vi "S2DS_Update Additional Info from user.vi"(11 "File info (in)":T1={"File path"=path "", "Header"="", "File name"="", "False channel"=[], "Channel names"=[], "Buffer size"=0, "Format"="%.6f"}) -> (2 "OK 2":bool, 3 "File info (out)":T1={"File path"=path "", "Header"="", "File name"="", "False channel"=[], "Channel names"=[], "Buffer size"=0, "Format"="%.6f"})   [LabVIEW 2025]
uses:
  TYPE DEFS/S2DS_Data saving info.ctl
panel:
  in  "CANCEL SWEEP":bool
  in  "Purpose":string
  in  "Skip":bool
  in  "OK":bool
  in  "False channel in (User)":string[][](array[string]) caption="Common information"
  # "Additional information"
  # "Information name"
  # "Value"
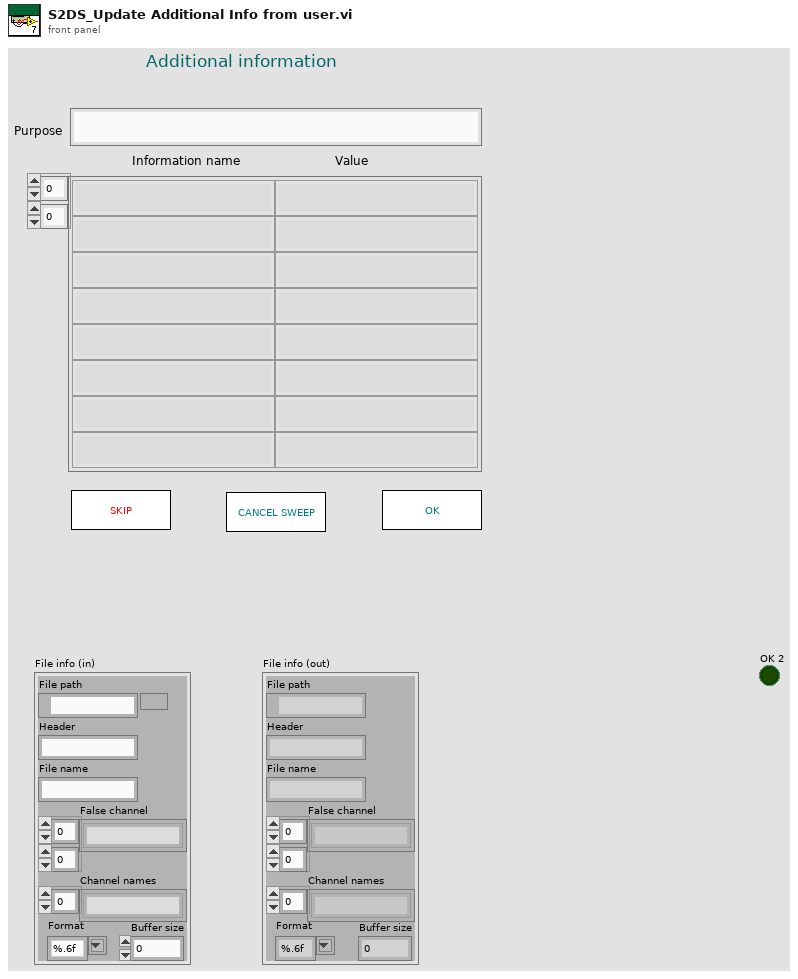
[diagram p1: front panel]
types:
  T1 = typedef "S2DS_Data saving info.ctl" = cluster{"File path":path, "Header":string, "File name":string, "False channel":string[][], "Channel names":string[], "Buffer size":i32, "Format":string}
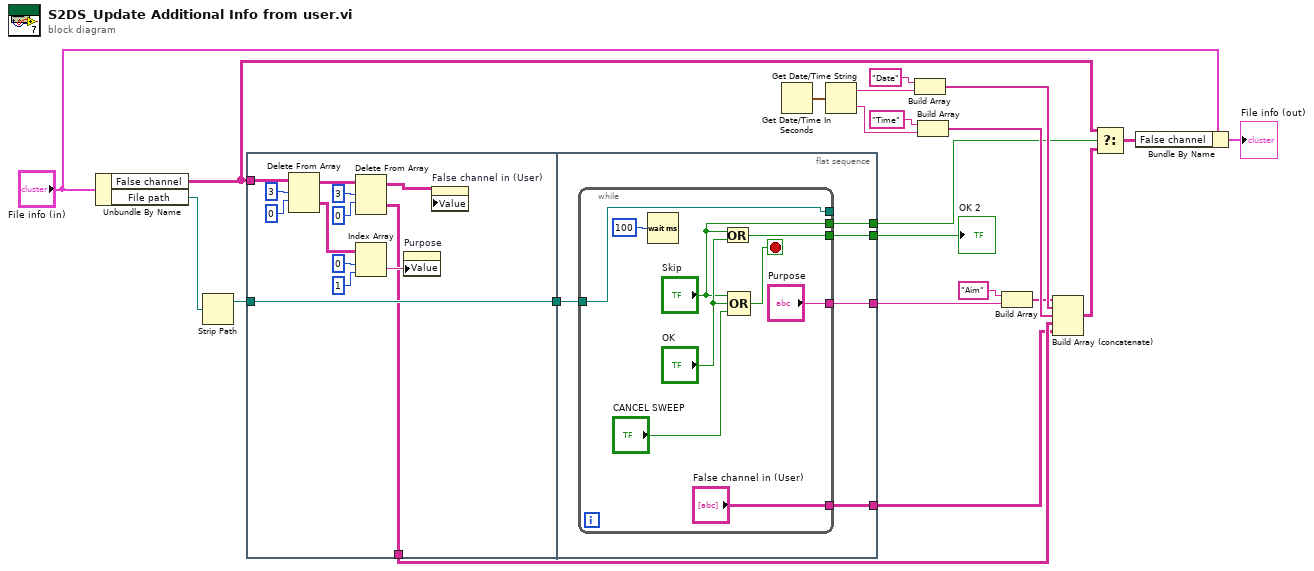
[diagram p0: block diagram]
diagram:
  n1 = Unbundle By Name("File info (in)") -> ("False channel"=w3:string[][], "File path"=w19:path)
  n2 = Strip Path(path=w19) -> (stripped path=w22:path)  [unwired: 1 out]
  n3 = flat-sequence {
    tunnel: w22 -> [w35]
    tunnel: [w35] -> w18
    tunnel: w3 -> [w34]
    tunnel: [w23] -> w6
    tunnel: [w39] -> w5
    tunnel: w18 -> [w40]
    tunnel: [w38] -> w17
    tunnel: [w37] -> w7
    tunnel: [w36] -> w4
    frame #0 {
      n4 = Delete From Array(array=w34, length=3, index (row)=0) -> (deleted portion=w31:string[][], array with subset deleted=w27:string[][])  [unwired: 1 in]
      n5 = Delete From Array(array=w27, length=3, index (row)=0) -> (deleted portion=w23:string[][], array with subset deleted=w24:string[][])  [unwired: 1 in]
      n6 = Index Array(array=w31, index (row)=0, index (col)=1 ("disabled index (col)")) -> (element=w28:string)
      n7 = property on="Purpose" class="Str"("Value"=w28) -> ()  [unwired: 2 in, 2 out]
      n8 = property on="False channel in (User)" class="Arr (strict)"("Value"=w24) -> ()  [unwired: 2 in, 2 out]
    }
    frame #1 {
      n9 = while {
        tunnel: ["False channel in (User)"] -> w39
        tunnel: [w47] -> _
        tunnel: w40 -> [w47]
        tunnel: [w43] -> w38
        tunnel: ["Purpose"] -> w37
        tunnel: ["Skip"] -> w36
        stop <- w45 stop-if-true
        n10 = Wait (ms)(milliseconds to wait=u32 100) -> ()  [unwired: 1 out]
        n11 = Or(x="Skip", y="OK") -> (x .or. y?=w43:bool)
        n12 = Compound Arithmetic op=OR("Skip", "OK", "CANCEL SWEEP") -> (w45:bool)
      }
    }
  }
  n13 = Get Date/Time In Seconds() -> (seconds since 1Jan1904=w16:timestamp)
  n14 = Get Date/Time String(seconds (now)=w16) -> (date string=w15:string, time string=w10:string)  [unwired: 2 in]
  n15 = Build Array("Date" ("element"), w15) -> (w12:string[])
  n16 = Build Array("Time" ("element"), w10) -> (w11:string[])
  n17 = Build Array("Aim" ("element"), w7) -> (w8:string[])
  n18 = Build Array (concatenate)(w8, w12, w11, w6, w5) -> (w2:string[][])
  n19 = Select(t=w3, s=w4, f=w2) -> (s? t:f=w1:string[][])
  n20 = Bundle By Name(cluster="File info (in)", "False channel"=w1) -> (→"File info (out)":T1)
  "OK 2" <- w17
